vi "RFC5322 Month String to Integer.vi"(11 "Month (string)":string) -> (3 "Month (Number)":i32)   [LabVIEW 2013]
uses:
  RFC5322 Months -- enum.ctl
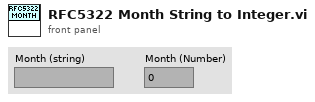
[diagram p1: front panel]
types:
  T1 = typedef "RFC5322 Months -- enum.ctl" = enum16{"Jan", "Feb", "Mar", "Apr", "May", "Jun", "Jul", "Aug", "Sep", "Oct", "Nov", "Dec"}
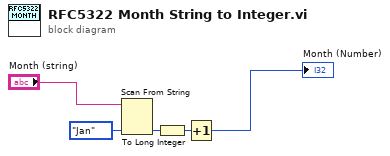
[diagram p0: block diagram]
diagram:
  n1 = Scan From String(input string="Month (string)", default 1=RFC5322_Months_--_enum."Jan") -> (output 1=w2:T1)  [unwired: 3 in, 3 out]
  n2 = To Long Integer(number=w2) -> (32bit integer=w1:i32)
  n3 = Increment(x=w1) -> (x+1=→"Month (Number)":i32)
